vi "Connect Report View.vi"(8 "error in (no error)":errorcluster, 11 "teststand-api in":refnum<class "teststand-api.lvclass">) -> (0 "error out":errorcluster, 3 "teststand-api out":refnum<class "teststand-api.lvclass">)   [LabVIEW 2014, in "teststand-api.lvlib" / "teststand-api.lvclass"]
uses:
  teststand-api.lvclass
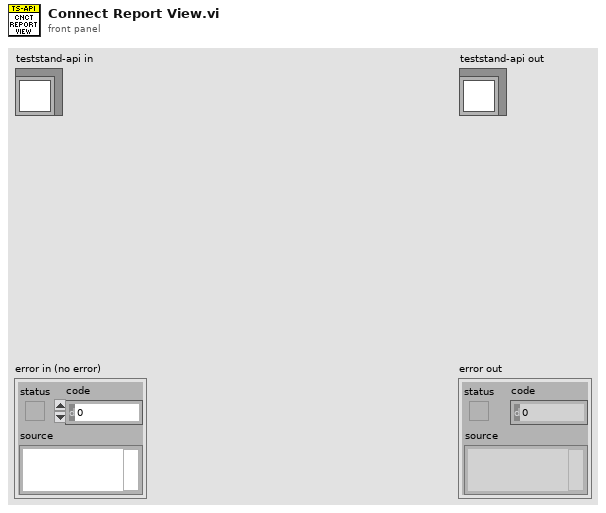
[diagram p1: front panel]
types:
  T1 = typedef "teststand-api.lvlib/teststand-api.lvclass/TS Controls Argument--cluster.ctl" = cluster{"Execution View":refnum<k7>, "Sequence View":refnum<k7>, "Report View":refnum<k7>}
  T2 = typedef "teststand-api.lvlib/teststand-api.lvclass/Manager Controls Argument--cluster.ctl" = cluster{"App Manager":refnum<k7>, "Seq Manager":refnum<k7>, "Exec Manager":refnum<k7>}
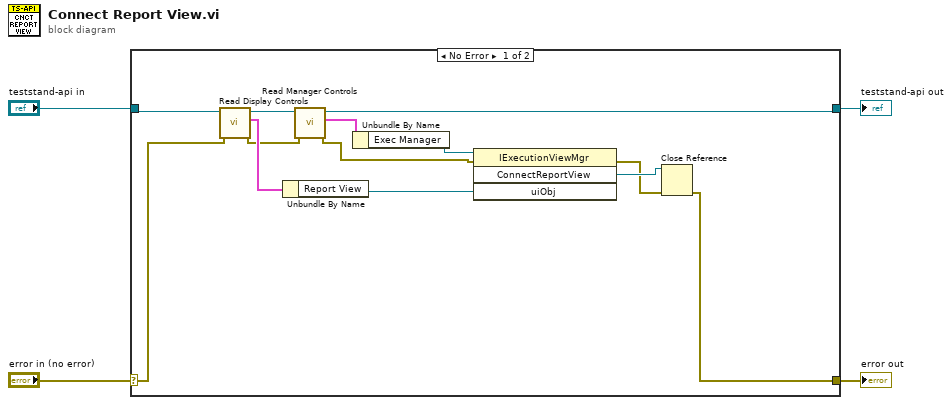
[diagram p0: block diagram]
diagram:
  n1 = case shown="No Error" "error in (no error)" {
    selector: "error in (no error)" -> [w5 w19]
    tunnel: [w7 w19] -> w3
    tunnel: [w17 w18] -> w1
    tunnel: "teststand-api in" -> [w13 w18]
    frame No Error {
      n2 = call-dynamic "Read Display Controls.vi"("error in (no error)"=w5, "teststand-api in"=w13) -> ("error out"=w11:errorcluster, "Visible Controls"=w12:T1, "teststand-api out"=w14:refnum<class "teststand-api.lvclass">)  [unwired: 7 in]
      n3 = Unbundle By Name(w12) -> ("Report View"=w10:refnum<k7>)
      n4 = call-dynamic "Read Manager Controls.vi"("error in (no error)"=w11, "teststand-api in"=w14) -> ("error out"=w6:errorcluster, "Manager Controls"=w16:T2, "teststand-api out"=w17:refnum<class "teststand-api.lvclass">)  [unwired: 7 in]
      n5 = Unbundle By Name(w16) -> ("Exec Manager"=w15:refnum<k7>)
      n6 = invoke class="IExecutionViewMgr" method="ConnectReportView"(reference=w15, error in=w6, "uiObj"=w10) -> (error out=w8:errorcluster, "ConnectReportView"=w9:refnum<k7>)  [unwired: 1 in, 2 out]
      n7 = Close Reference(reference=w9, error in (no error)=w8) -> (error out=w7:errorcluster)
    }
    frame Error {
    }
  }
  "error out" <- w3
  "teststand-api out" <- w1
